vi "Init App.vi"(8 "error in (no error)":errorcluster, 11 "VolatusCore in":refnum<class "VolatusCore.lvclass">) -> (0 "error out":errorcluster, 3 "VolatusCore out":refnum<class "VolatusCore.lvclass">)   [LabVIEW 2020, in "Volatus.lvlib" / "VolatusCore.lvclass"]
uses:
  VolatusCore.lvclass
  VolatusCore.lvclass/VolatusCore.ctl
  App/App.lvclass
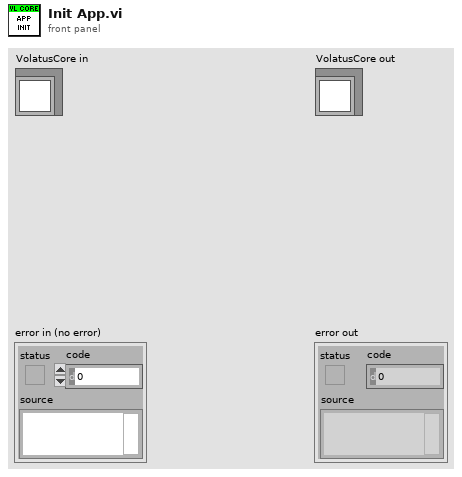
[diagram p1: front panel]
types:
  T1 = typedef "Volatus.lvlib/Core APIs.ctl" = cluster{"Volatus":refnum<class "VolatusAPI.lvclass">, "Event":refnum<class "EventAPI.lvclass">, "Telemetry":refnum<class "TelemetryAPI.lvclass">}
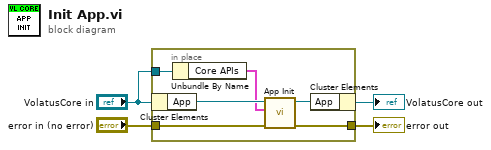
[diagram p0: block diagram]
diagram:
  n1 = in-place {
    in-place-border: "error in (no error)" -> [w10]
    in-place-border: [w9] -> w2
    in-place-border: "VolatusCore in" -> [w7]
    n2 = in-place-cluster #1("VolatusCore in") -> ("App"=w8:refnum<class "App.lvclass">)
    n3 = Unbundle By Name(w7) -> ("Core APIs"=w6:T1)
    n4 = call-dynamic "App Init.vi"("error in (no error)"=w10, "Core APIs"=w6, "App in"=w8) -> ("error out"=w9:errorcluster, "App out"=w5:refnum<class "App.lvclass">)  [unwired: 7 in]
    n5 = in-place-cluster #1("App"=w5) -> (→"VolatusCore out":refnum<class "VolatusCore.lvclass">)
  }
  "error out" <- w2
